vi "CmdexPwmFreq.vi"(8 "Uart Input":cluster{u64} {"?" format="%x"}, 10 "Frequency":sgl=50.0, 11 "Error Input":errorcluster) -> (0 "Uart Output":cluster{u64} {"?" format="%x"}, 3 "Error Output":errorcluster)   [LabVIEW 2019]
doc: "<B>Cmdex</B> \nChanges the frequency of all channels of PWM."
uses:
  dll/LabViewUart.dll
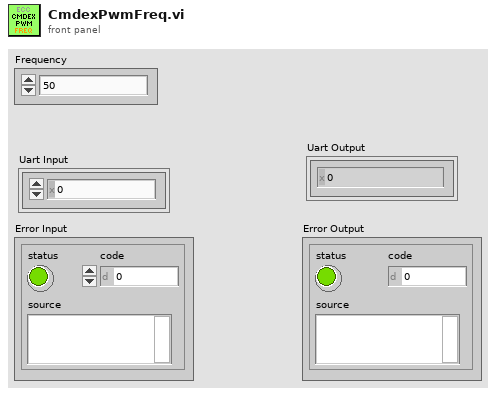
[diagram p1: front panel]
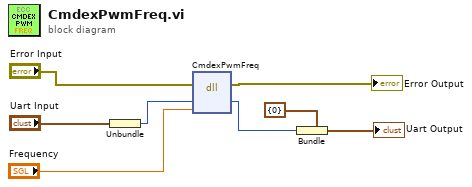
[diagram p0: block diagram]
diagram:
  n1 = Unbundle("Uart Input") -> (w5:u64)
  n2 = dll-call lib="D:/Google Drive/INC-2020/INC352/INC352-2020/LabVIEW/examples/uart-cmdex/SubVI/dll/LabViewUart.dll" fn="CmdexPwmFreq"(error in="Error Input", "Uart Handle"=w5, "frequency"="Frequency") -> (error out=→"Error Output":errorcluster, "Uart Handle"=w2:u64)  [unwired: 4 in, 1 out]
  n3 = Bundle(cluster=cluster{u64} {0}, w2) -> (→"Uart Output":cluster{u64})
